vi "Teleop.vi"(10 "Match Info":T1={"Autonomous Elapsed Seconds"=0.0, "TeleOp Elapsed Seconds"=0.0, "Disabled Elapsed Seconds"=0.0, "Visited Autonomous"=FALSE, "Visited TeleOp"=FALSE, "Visited Disabled"=FALSE, "Autonomous Settings"={"Autonomous Style"=enum."Independent", "VI Refnum"=refnum}}, 11 "Call Context":T2) -> ()   [LabVIEW 2013]
doc: "This VI is called for each TeleOp packet received from the DS where the robot is not disabled. It is often used to read from the joysticks and update I/O or to update setpoints for timed control loops. It should complete and return within 20 milliseconds or it may miss DS packets."
uses:
  <vilib>/Rock Robotics/WPI/DriverStation/WPI_DriverStationDerivedRobotMode.ctl
  <vilib>/Rock Robotics/WPI/DriverStation/WPI_DriverStationMatch Info.ctl
  Robot Global Data.vi
  <vilib>/Rock Robotics/WPI/Joystick/WPI_JoystickGetSetRefNum.vi
panel:
  in  "Slide":bool
  out "Numeric 1":dbl(slide) scale=0.0..100.0
  out "Boolean 2":bool
  out "Boolean 1":bool
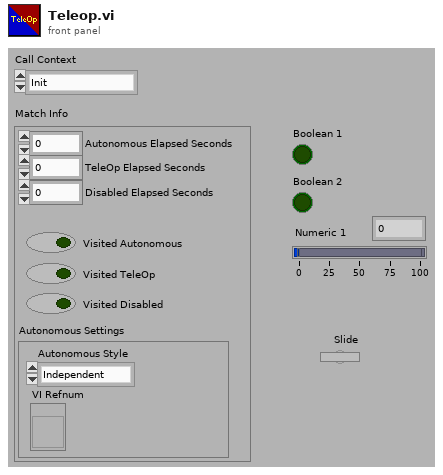
[diagram p1: front panel]
types:
  T1 = typedef "WPI_DriverStationMatch Info.ctl" = cluster{"Autonomous Elapsed Seconds":dbl, "TeleOp Elapsed Seconds":dbl, "Disabled Elapsed Seconds":dbl, "Visited Autonomous":bool, "Visited TeleOp":bool, "Visited Disabled":bool, "Autonomous Settings":cluster{"Autonomous Style":enum16{"Iterative", "Independent"}, "VI Refnum":refnum<vi>}}
  T2 = typedef "WPI_DriverStationDerivedRobotMode.ctl" = enum16{"Init", "Execute", "Stop"}
  T3 = typedef "WPI_JoystickDevRef.ctl" = cluster{"Device":T4}
  T4 = typedef "WPI_JoystickDeviceEnum.ctl" = enum16{"USB 1", "USB 2", "USB 3", "USB 4", "Kinect 1", "Kinect 2"}
  T5 = typedef "WPI_RobotDriveDevRef.ctl" = cluster{"DevStatus":errorcluster, "Motors[]":T6[], "Square Inputs":bool, "Max Output":dbl, "Isochronous":bool}
  T6 = typedef "WPI_MotorControlDeviceRef.ctl" = cluster{"DeviceStatus":errorcluster, "Type":enum16{"PWM", "CAN"}, "PWM":cluster{"Digital Module":T7, "PWM Channel":T8, "DeadBand":T9}, "CAN":cluster{"Device Number":u8, "Control Mode":T10, "Semaphore":T11, "Max Vout":dbl}, "Invert":bool, "TransformRef":T12, "InvTransformRef":T12}
  T7 = typedef "FPGA_TypedefDigitalModule.ctl" = enum16{"Digital Module 1", "Digital Module 2"}
  T8 = typedef "FPGA_DIOPWMChannel.ctl" = enum8{"PWM 1", "PWM 2", "PWM 3", "PWM 4", "PWM 5", "PWM 6", "PWM 7", "PWM 8", "PWM 9", "PWM 10", "Invalid"}
  T9 = typedef "WPI_PWMDeadband.ctl" = cluster{"Name":string, "maxPositivePwm":i32, "minPositivePwm":i32, "centerPwm":i32, "maxNegativePwm":i32, "minNegativePwm":i32, "angularRange":u16}
  T10 = typedef "WPI_CANJaguar_ControlMode.ctl" = enum8{"Percent VBus", "Current", "Speed", "Position", "Voltage"}
  T11 = typedef "Semaphore RefNum" = refnum<k1>
  T12 = typedef "WPI_PWMTransform_ConPane.ctl" = refnum<vi>
  T13 = typedef "WPI_JoystickButtonState.ctl" = cluster{"Button 1":bool, "Button 2":bool, "Button 3":bool, "Button 4":bool, "Button 5":bool, "Button 6":bool, "Button 7":bool, "Button 8":bool, "Button 9":bool, "Button 10":bool, "Button 11":bool, "Button 12":bool}
  T14 = cluster{"axis 1 (x)":dbl, "axis 2 (y)":dbl, "axis 3 (throttle)":dbl, "axis 4":dbl, "axis 5":dbl, "axis 6":dbl}
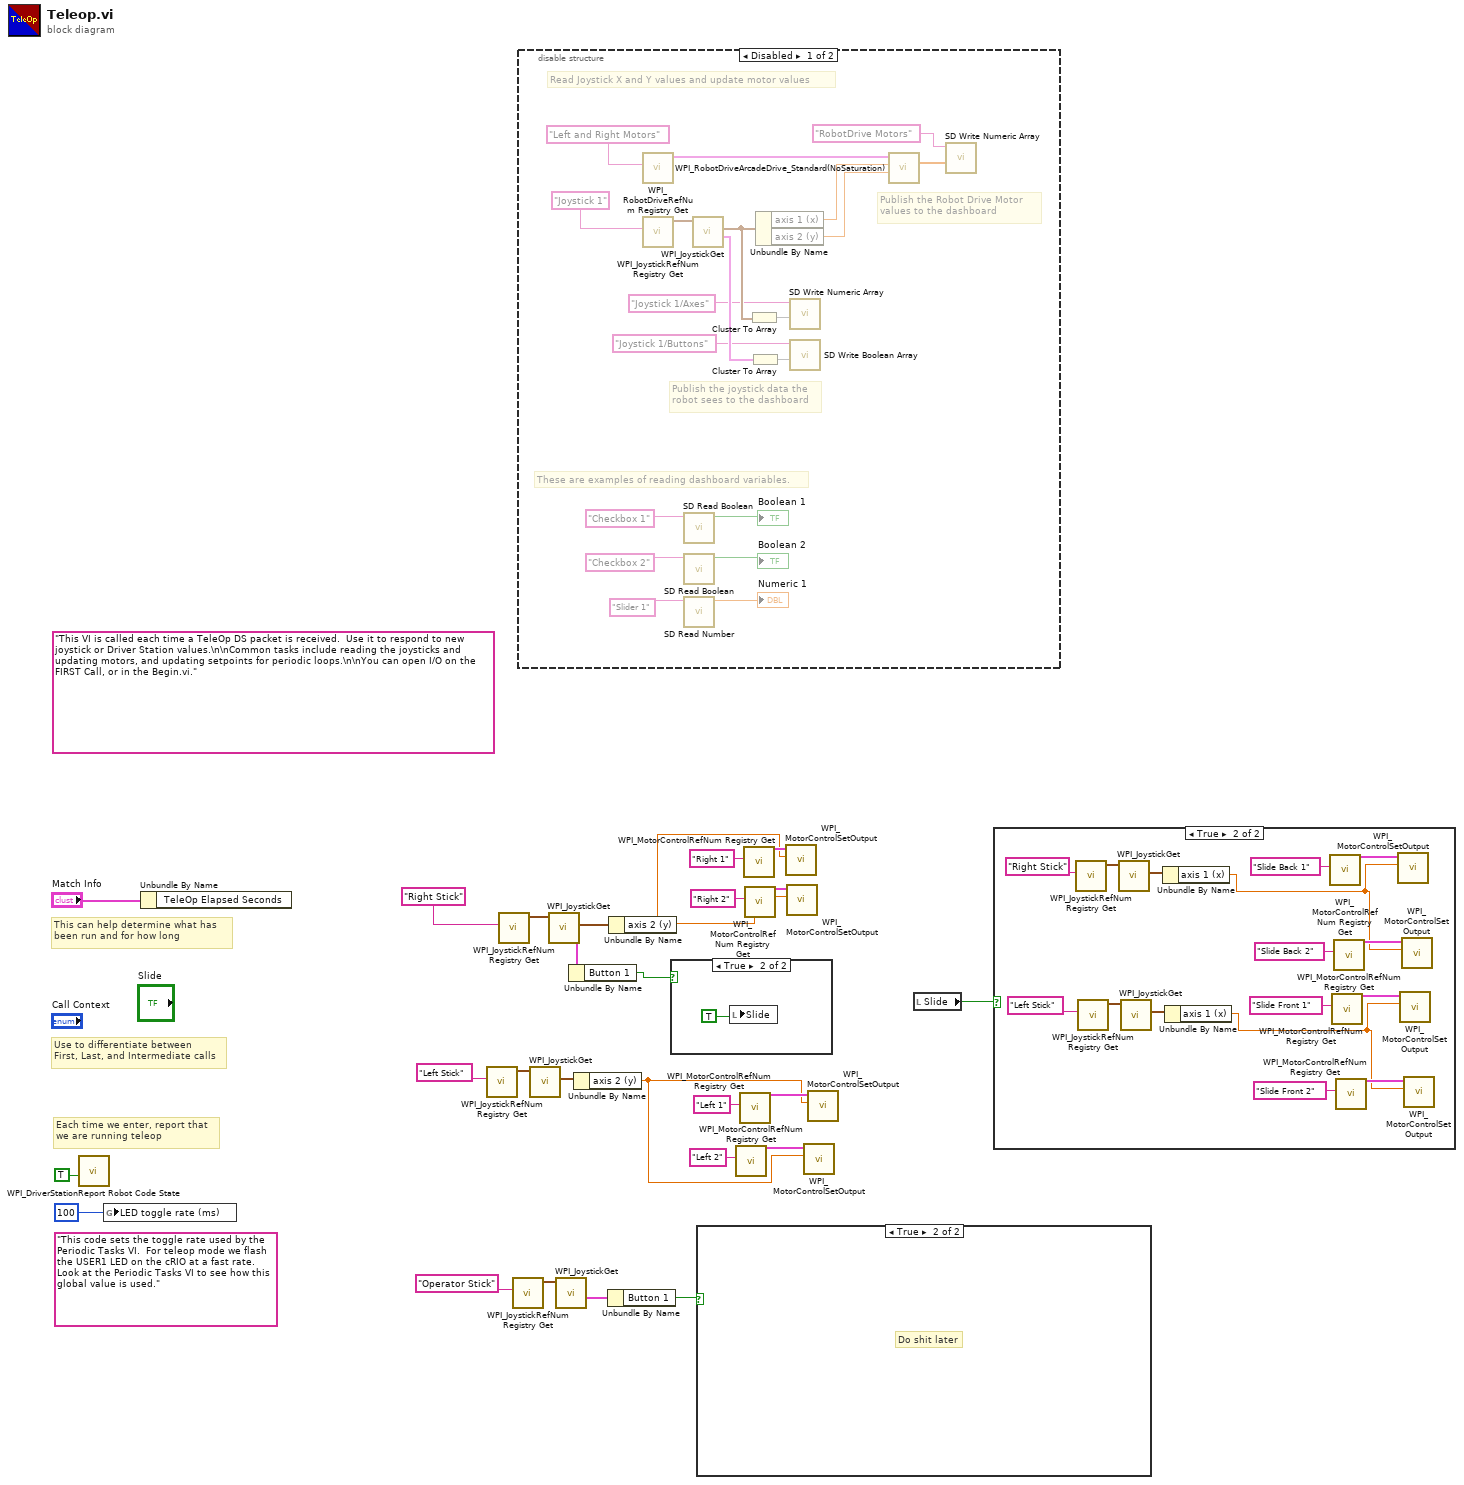
[diagram p0: block diagram]
diagram:
  (unwired) "This code sets the toggle rate used by the Periodic Tasks VI.  For teleop mode we flash the USER1 LED on the cRIO at a fast rate.  Look at the Periodic Tasks VI to see how this global value is used."
  (unwired) "This VI is called each time a TeleOp DS packet is received.  Use it to respond to new joystick or Driver Station values.\n\nCommon tasks include reading the joysticks and updating motors, and updating setpoints for periodic loops.\n\nYou can open I/O on the FIRST Call, or in the Begin.vi."
  # "Each time we enter, report that\nwe are running teleop"
  # "Use to differentiate between\nFirst, Last, and Intermediate calls"
  # "This can help determine what has\nbeen run and for how long"
  n1 = call <vilib>:"WPI_DriverStationReport Robot Code State.vi"("TeleOp"=TRUE ("Autonomous")) -> ()  [unwired: 10 in, 1 out]
  n2 = global write "Robot Global Data.vi" "LED toggle rate (ms)"(u32 100 ("LED ms toggle rate")) -> ()
  n3 = Unbundle By Name("Match Info") -> ()  [unwired: 1 out]
  n4 = call <vilib>:"WPI_JoystickRefNum Registry Get.vi"("refnum name"="Left Stick") -> ("JoystickDevRef"=w23:T3)  [unwired: 9 in, 1 out]
  n5 = call <vilib>:"WPI_JoystickRefNum Registry Get.vi"("refnum name"="Right Stick") -> ("JoystickDevRef"=w20:T3)  [unwired: 1 in, 9 out]
  n6 = call <vilib>:"WPI_JoystickRefNum Registry Get.vi"("refnum name"="Operator Stick") -> ("JoystickDevRef"=w4:T3)  [unwired: 9 in, 1 out]
  n7 = disable-structure shown="Disabled" {
    frame Disabled {
      # "Publish the Robot Drive Motor\nvalues to the dashboard"
      # "These are examples of reading dashboard variables."
      # "Publish the joystick data the\nrobot sees to the dashboard"
      # "Read Joystick X and Y values and update motor values"
      n8 = call <vilib>:"WPI_RobotDriveRefNum Registry Get.vi"("refnum name"="Left and Right Motors") -> ("RobotDriveDevRef"=w45:T5)  [unwired: 1 in, 9 out]
      n9 = call <vilib>:"WPI_JoystickRefNum Registry Get.vi"("refnum name"="Joystick 1") -> ("JoystickDevRef"=w41:T3)  [unwired: 1 in, 9 out]
      n10 = call <vilib>:"SD Read Boolean.vi"("Name"="Checkbox 1" ("refnum name")) -> ("Boolean"=→"Boolean 1":bool)  [unwired: 8 in, 2 out]
      n11 = call <vilib>:"SD Read Boolean.vi"("Name"="Checkbox 2" ("refnum name")) -> ("Boolean"=→"Boolean 2":bool)  [unwired: 8 in, 2 out]
      n12 = call <vilib>:"SD Read Number.vi"("Name"="Slider 1" ("refnum name")) -> ("Numeric"=→"Numeric 1":dbl)  [unwired: 8 in, 2 out]
      n13 = call <vilib>:"WPI_JoystickGet.vi"("JoystickDevRef"=w41) -> ("Buttons"=w40:T13, "Axes"=w37:T14)  [unwired: 1 in, 4 out]
      n14 = Cluster To Array(cluster=w37) -> (array=w36:dbl[])
      n15 = Cluster To Array(cluster=w40) -> (array=w39:bool[])
      n16 = Unbundle By Name(w37) -> ("axis 1 (x)"=w44:dbl, "axis 2 (y)"=w43:dbl)
      n17 = call <vilib>:"SD Write Numeric Array.vi"("Numeric Array"=w36, "Name"="Joystick 1/Axes") -> ()  [unwired: 8 in, 2 out]
      n18 = call <vilib>:"SD Write Boolean Array.vi"("Boolean Array"=w39, "Name"="Joystick 1/Buttons") -> ()  [unwired: 8 in, 2 out]
      n19 = call <vilib>:"WPI_RobotDriveArcadeDrive_Standard(NoSaturation).vi"("Y axis value"=w43, "X axis value"=w44, "RobotDriveDevRef"=w45) -> ("Motor Values"=w33:dbl[])  [unwired: 1 in, 7 out]
      n20 = call <vilib>:"SD Write Numeric Array.vi"("Numeric Array"=w33, "Name"="RobotDrive Motors") -> ()  [unwired: 8 in, 2 out]
    }
    frame Enabled {
    }
  }
  n21 = call <vilib>:"WPI_JoystickGet.vi"("JoystickDevRef"=w23) -> ("Axes"=w8:T14)  [unwired: 4 in, 2 out]
  n22 = call <vilib>:"WPI_JoystickGet.vi"("JoystickDevRef"=w20) -> ("Buttons"=w7:T13, "Axes"=w19:T14)  [unwired: 1 in, 4 out]
  n23 = call <vilib>:"WPI_JoystickGet.vi"("JoystickDevRef"=w4) -> ("Buttons"=w2:T13)  [unwired: 4 in, 2 out]
  n24 = Unbundle By Name(w7) -> ("Button 1"=w6:bool)
  n25 = Unbundle By Name(w8) -> ("axis 2 (y)"=w9:dbl)
  n26 = Unbundle By Name(w2) -> ("Button 1"=w1:bool)
  n27 = Unbundle By Name(w19) -> ("axis 2 (y)"=w14:dbl)
  n28 = case shown="True" w6 {
    frame False {
    }
    frame True {
      n29 = local write "Slide"(TRUE) -> ()
    }
  }
  n30 = case shown="True" w1 {
    frame False {
    }
    frame True {
      # "Do shit later"
    }
  }
  n31 = call <vilib>:"WPI_MotorControlRefNum Registry Get.vi"("refnum name"="Left 2") -> ("MotorControlDevRef"=w10:T6)  [unwired: 9 in, 1 out]
  n32 = call <vilib>:"WPI_MotorControlRefNum Registry Get.vi"("refnum name"="Left 1") -> ("MotorControlDevRef"=w12:T6)  [unwired: 9 in, 1 out]
  n33 = call <vilib>:"WPI_MotorControlRefNum Registry Get.vi"("refnum name"="Right 1") -> ("MotorControlDevRef"=w17:T6)  [unwired: 9 in, 1 out]
  n34 = call <vilib>:"WPI_MotorControlRefNum Registry Get.vi"("refnum name"="Right 2") -> ("MotorControlDevRef"=w15:T6)  [unwired: 9 in, 1 out]
  n35 = call <vilib>:"WPI_MotorControlSetOutput.vi"("Output"=w14, "MotorControlDevRef"=w17) -> ()  [unwired: 7 in, 3 out]
  n36 = call <vilib>:"WPI_MotorControlSetOutput.vi"("Output"=w14, "MotorControlDevRef"=w15) -> ()  [unwired: 7 in, 3 out]
  n37 = call <vilib>:"WPI_MotorControlSetOutput.vi"("Output"=w9, "MotorControlDevRef"=w10) -> ()  [unwired: 7 in, 3 out]
  n38 = call <vilib>:"WPI_MotorControlSetOutput.vi"("Output"=w9, "MotorControlDevRef"=w12) -> ()  [unwired: 7 in, 3 out]
  n39 = local read "Slide"() -> (w5:bool)
  n40 = case shown="True" w5 {
    frame False {
    }
    frame True {
      n41 = call <vilib>:"WPI_JoystickRefNum Registry Get.vi"("refnum name"="Right Stick") -> ("JoystickDevRef"=w55:T3)  [unwired: 9 in, 1 out]
      n42 = call <vilib>:"WPI_JoystickRefNum Registry Get.vi"("refnum name"="Left Stick") -> ("JoystickDevRef"=w63:T3)  [unwired: 9 in, 1 out]
      n43 = call <vilib>:"WPI_JoystickGet.vi"("JoystickDevRef"=w55) -> ("Axes"=w53:T14)  [unwired: 4 in, 2 out]
      n44 = call <vilib>:"WPI_JoystickGet.vi"("JoystickDevRef"=w63) -> ("Axes"=w61:T14)  [unwired: 4 in, 2 out]
      n45 = Unbundle By Name(w53) -> ("axis 1 (x)"=w48:dbl)
      n46 = Unbundle By Name(w61) -> ("axis 1 (x)"=w56:dbl)
      n47 = call <vilib>:"WPI_MotorControlRefNum Registry Get.vi"("refnum name"="Slide Back 1") -> ("MotorControlDevRef"=w51:T6)  [unwired: 9 in, 1 out]
      n48 = call <vilib>:"WPI_MotorControlRefNum Registry Get.vi"("refnum name"="Slide Front 1") -> ("MotorControlDevRef"=w59:T6)  [unwired: 9 in, 1 out]
      n49 = call <vilib>:"WPI_MotorControlRefNum Registry Get.vi"("refnum name"="Slide Back 2") -> ("MotorControlDevRef"=w49:T6)  [unwired: 9 in, 1 out]
      n50 = call <vilib>:"WPI_MotorControlRefNum Registry Get.vi"("refnum name"="Slide Front 2") -> ("MotorControlDevRef"=w57:T6)  [unwired: 9 in, 1 out]
      n51 = call <vilib>:"WPI_MotorControlSetOutput.vi"("Output"=w48, "MotorControlDevRef"=w51) -> ()  [unwired: 7 in, 3 out]
      n52 = call <vilib>:"WPI_MotorControlSetOutput.vi"("Output"=w56, "MotorControlDevRef"=w59) -> ()  [unwired: 7 in, 3 out]
      n53 = call <vilib>:"WPI_MotorControlSetOutput.vi"("Output"=w48, "MotorControlDevRef"=w49) -> ()  [unwired: 7 in, 3 out]
      n54 = call <vilib>:"WPI_MotorControlSetOutput.vi"("Output"=w56, "MotorControlDevRef"=w57) -> ()  [unwired: 7 in, 3 out]
    }
  }
